vi "loadRFRampData.vi"(8 "error in (no error)":errorcluster, 10 "RfRamp":refnum<class "RfRamp.lvclass">, 11 "Rf_Ramp_Action in":refnum<class "Rf_Ramp_Action.lvclass">) -> (0 "error out":errorcluster, 2 "RfRamp out":refnum<class "RfRamp.lvclass">, 3 "Rf_Ramp_Action out":refnum<class "Rf_Ramp_Action.lvclass">)   [LabVIEW 2011, in "Views.lvlib" / "ScriptEditor.lvlib" / "Rf_Ramp_Action.lvclass"]
uses:
  Rf_Ramp_Action.lvclass
  Tools/Scripting/ScriptingEvent/ScriptEvents/RfRamp/RfRamp.lvclass
  Rf_Ramp_Action.lvclass/Rf_Ramp_Action.ctl
  Tools/Scripting/ScriptingEvent/ScriptEvents/Rf Event/rf.lvclass
  Tools/Scripting/ScriptingEvent/ScriptEvent.lvclass
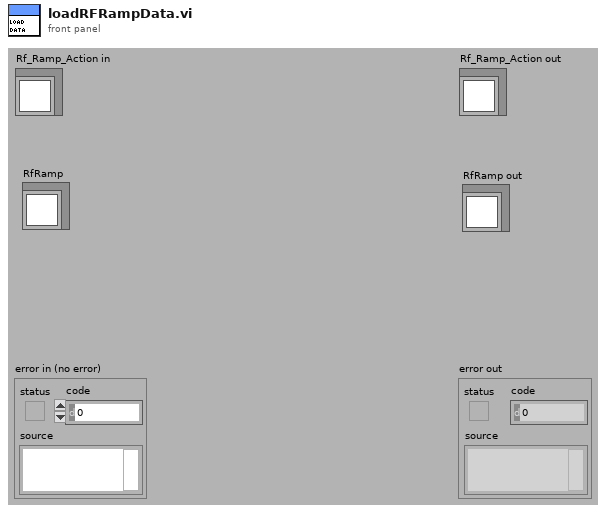
[diagram p1: front panel]
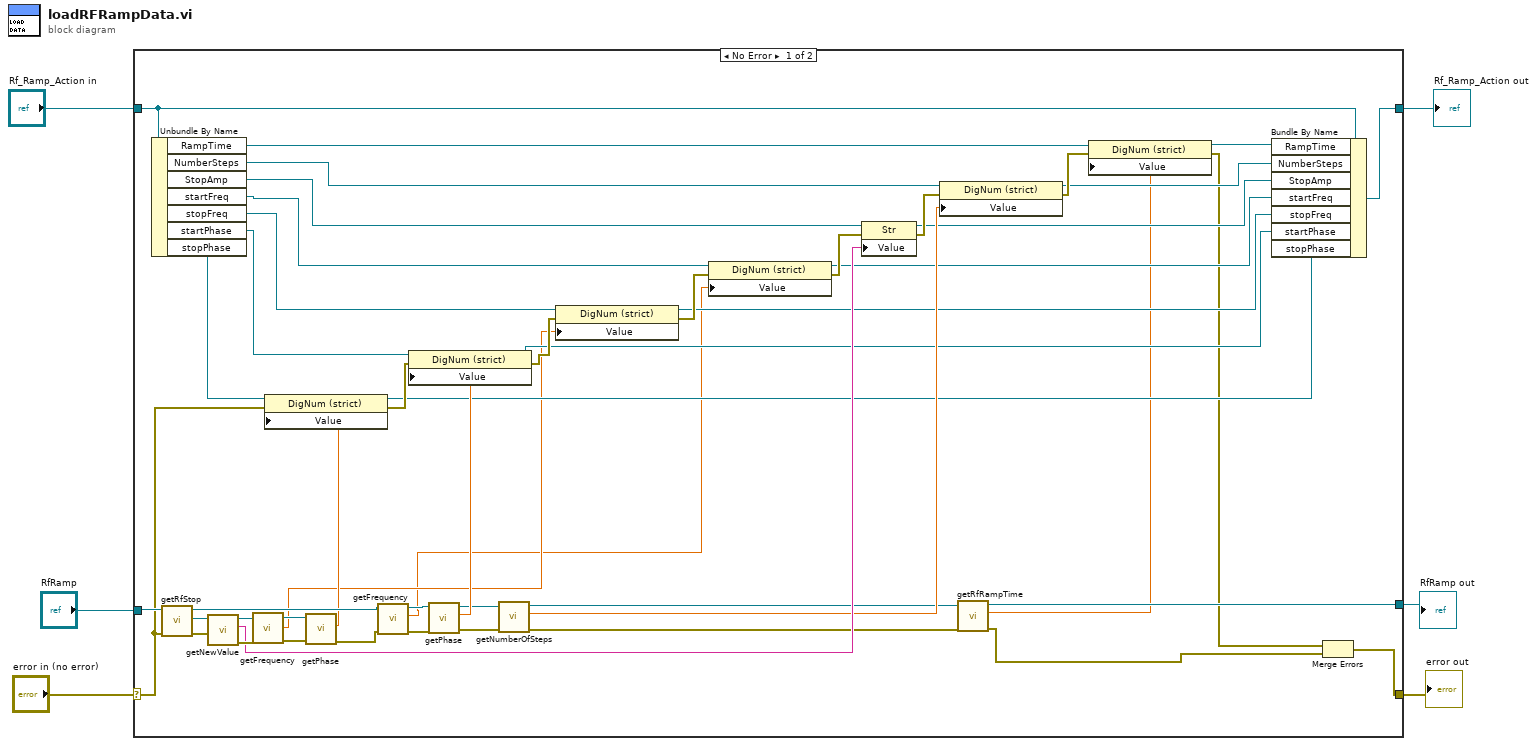
[diagram p0: block diagram]
diagram:
  n1 = case shown="No Error" "error in (no error)" {
    selector: "error in (no error)" -> [w42 w58]
    tunnel: [w10 w58] -> w5
    tunnel: [w15 w57] -> w3
    tunnel: "Rf_Ramp_Action in" -> [w16 w57]
    tunnel: "RfRamp" -> [w53 w56]
    tunnel: [w13 w56] -> w1
    frame No Error {
      n2 = Unbundle By Name(w16) -> ("RampTime"=w24:refnum<vi>, "NumberSteps"=w29:refnum<vi>, "StopAmp"=w34:refnum<vi>, "startFreq"=w36:refnum<vi>, "stopFreq"=w39:refnum<vi>, "startPhase"=w54:refnum<vi>, "stopPhase"=w55:refnum<vi>)
      n3 = call "getRfStop.vi"("error in (no error)"=w42, "RfRamp in"=w53) -> ("error out"=w45:errorcluster, "rfStop"=w46:refnum<class "rf.lvclass">, "RfRamp out"=w50:refnum<class "RfRamp.lvclass">)  [unwired: 7 in]
      n4 = call "getNewValue.vi"("error in (no error)"=w45, "ScriptEvent.lvclass in"=w46) -> ("error out"=w44:errorcluster, "newValue"=w33:string, "ScriptEvent.lvclass out"=w47:refnum<class "rf.lvclass">)  [unwired: 7 in]
      n5 = call "getFrequency.vi"("error in (no error)"=w44, "rf in"=w47) -> ("error out"=w48:errorcluster, "frequency"=w8:dbl, "rf out"=w52:refnum<class "rf.lvclass">)  [unwired: 7 in]
      n6 = call "getPhase.vi"("error in (no error)"=w48, "rf in"=w52) -> ("error out"=w49:errorcluster, "phase"=w41:dbl)  [unwired: 7 in, 1 out]
      n7 = property class="DigNum (strict)"(reference=w55, error in=w42, "Value"=w41) -> (reference out=w14:refnum<vi>, error out=w17:errorcluster)
      n8 = call "getFrequency.vi"("error in (no error)"=w49, "rf in"=w50) -> ("error out"=w43:errorcluster, "frequency"=w7:dbl, "rf out"=w51:refnum<class "RfRamp.lvclass">)  [unwired: 7 in]
      n9 = call "getPhase.vi"("error in (no error)"=w43, "rf in"=w51) -> ("error out"=w31:errorcluster, "phase"=w40:dbl, "rf out"=w32:refnum<class "RfRamp.lvclass">)  [unwired: 7 in]
      n10 = property class="DigNum (strict)"(reference=w54, error in=w17, "Value"=w40) -> (reference out=w18:refnum<vi>, error out=w38:errorcluster)
      n11 = call "getNumberOfSteps.vi"("error in (no error)"=w31, "RfRamp in"=w32) -> ("error out"=w26:errorcluster, "NumberOfSteps"=w28:dbl, "RfRamp out"=w27:refnum<class "RfRamp.lvclass">)  [unwired: 7 in]
      n12 = property class="DigNum (strict)"(reference=w39, error in=w38, "Value"=w8) -> (reference out=w19:refnum<vi>, error out=w37:errorcluster)
      n13 = property class="DigNum (strict)"(reference=w36, error in=w37, "Value"=w7) -> (reference out=w20:refnum<vi>, error out=w35:errorcluster)
      n14 = property class="Str"(reference=w34, error in=w35, "Value"=w33) -> (reference out=w21:refnum<vi>, error out=w30:errorcluster)
      n15 = property class="DigNum (strict)"(reference=w29, error in=w30, "Value"=w28) -> (reference out=w22:refnum<vi>, error out=w25:errorcluster)
      n16 = call "getRfRampTime.vi"("error in (no error)"=w26, "RfRamp in"=w27) -> ("error out"=w11:errorcluster, "rampTime"=w9:dbl, "RfRamp out"=w13:refnum<class "RfRamp.lvclass">)  [unwired: 7 in]
      n17 = property class="DigNum (strict)"(reference=w24, error in=w25, "Value"=w9) -> (reference out=w23:refnum<vi>, error out=w12:errorcluster)
      n18 = Bundle By Name(cluster=w16, "RampTime"=w23, "NumberSteps"=w22, "StopAmp"=w21, "startFreq"=w20, "stopFreq"=w19, "startPhase"=w18, "stopPhase"=w14) -> (w15:refnum<class "Rf_Ramp_Action.lvclass">)
      n19 = Merge Errors(w12, w11) -> (w10:errorcluster)
    }
    frame Error {
    }
  }
  "error out" <- w5
  "Rf_Ramp_Action out" <- w3
  "RfRamp out" <- w1
